vi "cornell-K0edges.vi"(6 "Numeric":i32=500, 7 "secelt":T1, 8 "τ":dbl=1.0, 9 "h":dbl, 10 "s":dbl, 11 "ω":dbl) -> (0 "Ks(ω)":cdb)   [LabVIEW 2020]
uses:
  cornell-Ktildesh2sides.ctl
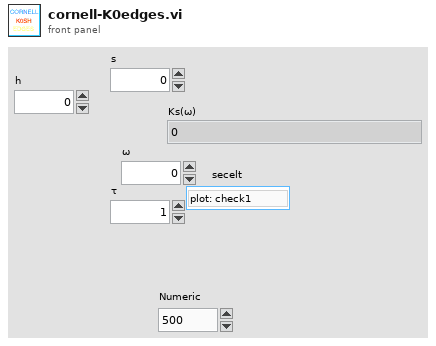
[diagram p1: front panel]
types:
  T1 = typedef "cornell-Ktildesh2sides.ctl" = enum16{"plot: check1", "plot: check2", "plot: one½", "plot: two½", "plot: uni½", "calc: zcoth(z)", "calc: z/sinh(z)", "calc: brute", "calc: integra", "void", "plot: nano"}
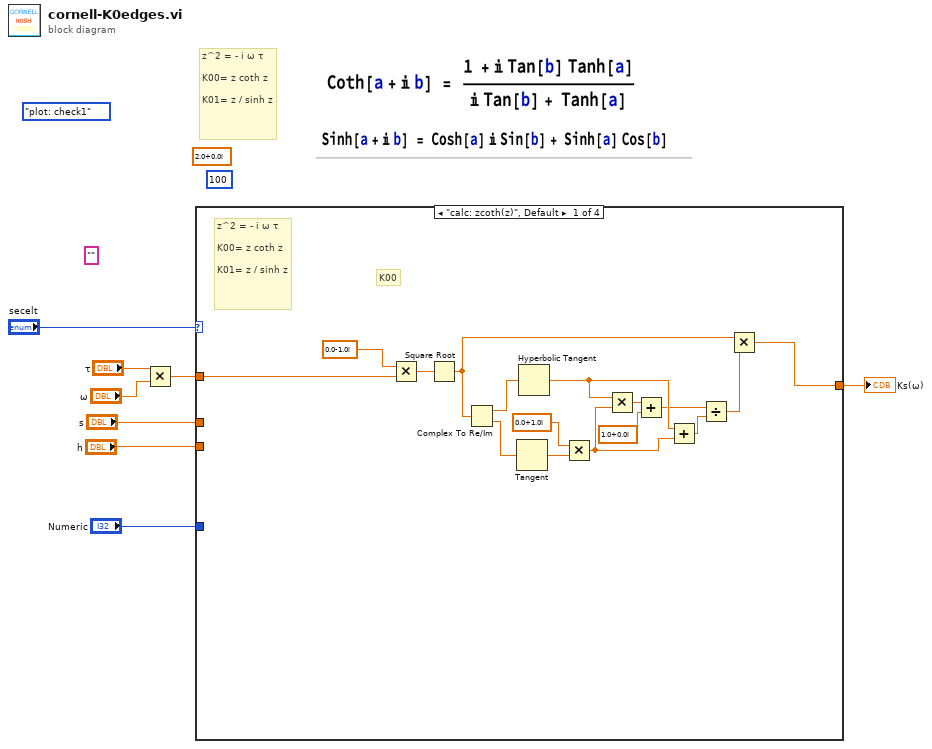
[diagram p0: block diagram]
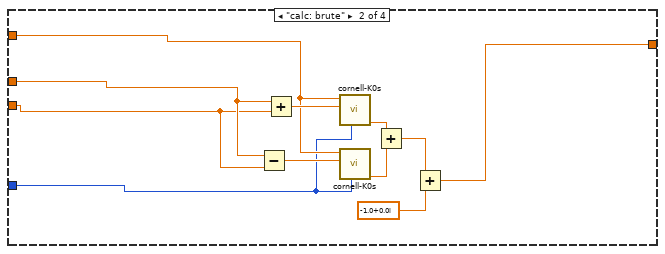
[diagram p2: hidden frame]
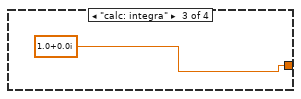
[diagram p3: hidden frame]
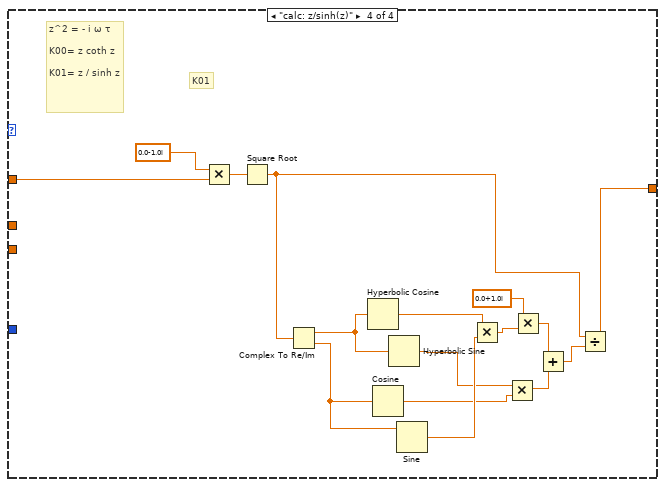
[diagram p4: hidden frame]
diagram:
  (unwired) cornell-Ktildesh2sides."plot: check1" ("Enum")
  (unwired) ""
  (unwired) cdb 2.0+0.0i
  (unwired) 100
  # "z^2 = - i ω τ\n\nK00= z coth z\n\nK01= z / sinh z"
  n1 = Multiply(x="τ", y="ω") -> (x*y=w4:dbl)
  n2 = case shown="\"calc: zcoth(z)\", Default" "secelt" {
    tunnel: "s" -> [_ w28 _ _]
    tunnel: "h" -> [_ w27 _ _]
    tunnel: w4 -> [w24 w29 _ w52]
    tunnel: [w9 w25 cdb 1.0+0.0i ("s") w37] -> w3
    tunnel: "Numeric" -> [_ w26 _ _]
    frame "calc: zcoth(z)", Default {
      # "K00"
      # "z^2 = - i ω τ\n\nK00= z coth z\n\nK01= z / sinh z"
      n3 = Multiply(x=cdb 0.0-1.0i, y=w24) -> (x*y=w22:cdb)
      n4 = Square Root(x=w22) -> (sqrt(x)=w10:cdb)
      n5 = Complex To Re/Im(x + iy=w10) -> (x=w19:dbl, y=w18:dbl)
      n6 = Tangent(1:w18) -> (0:w21:dbl)
      n7 = Hyperbolic Tangent(1:w19) -> (0:w15:dbl)
      n8 = Multiply(x=cdb 0.0+1.0i, y=w21) -> (x*y=w14:cdb)
      n9 = Multiply(x=w15, y=w14) -> (x*y=w17:cdb)
      n10 = Add(x=w17, y=cdb 1.0+0.0i) -> (x+y=w12:cdb)
      n11 = Add(x=w15, y=w14) -> (x+y=w13:cdb)
      n12 = Divide(x=w12, y=w13) -> (x/y=w11:cdb)
      n13 = Multiply(x=w10, y=w11) -> (x*y=w9:cdb)
    }
    frame "calc: brute" {
      n14 = Subtract(x=w28, y=w27) -> (x-y=w34:dbl)
      n15 = Add(x=w28, y=w27) -> (x+y=w35:dbl)
      n16 = call "cornell-K0s.vi"("Numeric"=w26, "s"=w35, "ω"=w29) -> ("Ks(ω)"=w33:cdb)  [unwired: 8 in]
      n17 = call "cornell-K0s.vi"("Numeric"=w26, "s"=w34, "ω"=w29) -> ("Ks(ω)"=w32:cdb)  [unwired: 8 in]
      n18 = Add(x=w33, y=w32) -> (x+y=w31:cdb)
      n19 = Add(x=w31, y=cdb -1.0+0.0i ("x")) -> (x+y=w25:cdb)
    }
    frame "calc: integra" {
    }
    frame "calc: z/sinh(z)" {
      # "K01"
      # "z^2 = - i ω τ\n\nK00= z coth z\n\nK01= z / sinh z"
      n20 = Multiply(x=cdb 0.0-1.0i, y=w52) -> (x*y=w50:cdb)
      n21 = Square Root(x=w50) -> (sqrt(x)=w39:cdb)
      n22 = Complex To Re/Im(x + iy=w39) -> (x=w49:dbl, y=w48:dbl)
      n23 = Hyperbolic Cosine(1:w49) -> (0:w47:dbl)
      n24 = Cosine(x=w48) -> (cos(x)=w42:dbl)
      n25 = Hyperbolic Sine(1:w49) -> (0:w43:dbl)
      n26 = Sine(x=w48) -> (sin(x)=w46:dbl)
      n27 = Multiply(x=w47, y=w46) -> (x*y=w44:dbl)
      n28 = Multiply(x=w43, y=w42) -> (x*y=w40:dbl)
      n29 = Multiply(x=cdb 0.0+1.0i, y=w44) -> (x*y=w41:cdb)
      n30 = Add(x=w41, y=w40) -> (x+y=w38:cdb)
      n31 = Divide(x=w39, y=w38) -> (x/y=w37:cdb)
    }
  }
  "Ks(ω)" <- w3
